vi "Day 2 - Rock Paper Scissors.vi"() -> ()   [LabVIEW 2020, in "AoC 2022.lvlib"]
uses:
  AoC 2022.lvlib
panel:
  out "Puzzle Part-2 Answer":string
  out "Puzzle Answer":string
  in  "Puzzle Input":string
  # "Enter the Puzzle Input and run the VI"
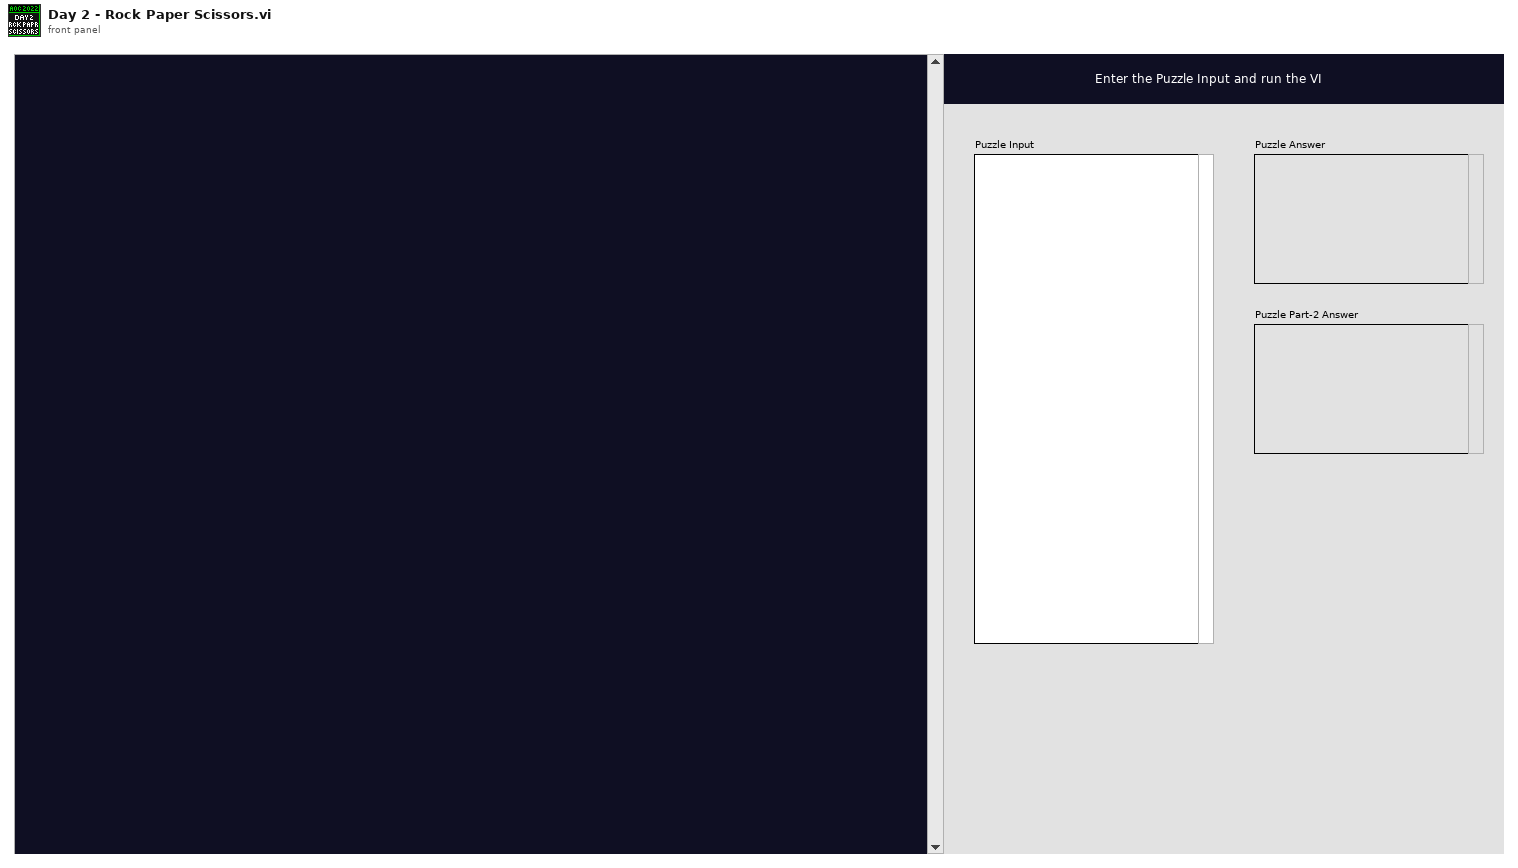
[diagram p1: front panel]
types:
  T1 = typedef "AoC 2022.lvlib/Play Item.ctl" = enum16{"Rock", "Paper", "Scissor"}
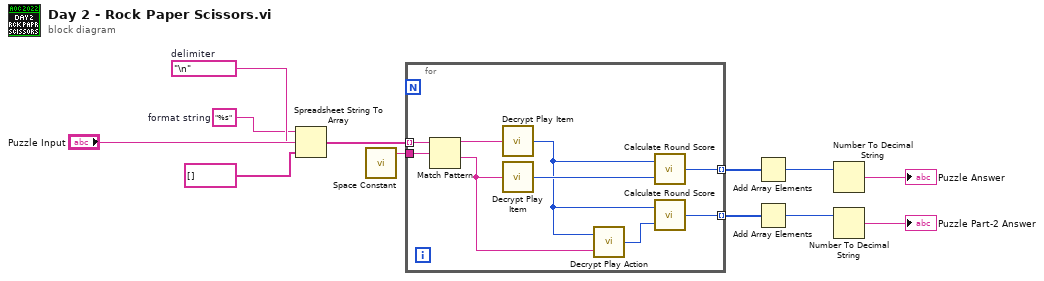
[diagram p0: block diagram]
diagram:
  w10 = "%s"  # format string
  w11 = "\n"  # delimiter
  n1 = Spreadsheet String To Array(delimiter (Tab)=w11, format string=w10, spreadsheet string="Puzzle Input", array type (2D Dbl)=string[] []) -> (array=w8:string[])
  n2 = call <vilib>:"Space Constant.vi"() -> ("String"=w7:string)
  n3 = for {
    tunnel: w8 -> [w21] mode=indexing
    tunnel: w7 -> [w20]
    tunnel: [w17] -> w6 mode=indexing
    tunnel: [w13] -> w2 mode=indexing
    n4 = Match Pattern(string=w21, regular expression=w20) -> (before substring=w19:string, after substring=w16:string)  [unwired: 1 in, 2 out]
    n5 = call "Decrypt Play Item.vi"("Encrypted Play Item"=w19) -> ("Play Item"=w15:T1)  [unwired: 4 in]
    n6 = call "Decrypt Play Item.vi"("Encrypted Play Item"=w16) -> ("Play Item"=w18:T1)  [unwired: 4 in]
    n7 = call "Decrypt Play Action.vi"("Encrypted Play Action"=w16, "Opponent's Move"=w15) -> ("My Move"=w14:T1)
    n8 = call "Calculate Round Score.vi"("My Move"=w18, "Opponent's Move"=w15) -> ("Round Score"=w17:u32)
    n9 = call "Calculate Round Score.vi"("My Move"=w14, "Opponent's Move"=w15) -> ("Round Score"=w13:u32)
  }
  n10 = Add Array Elements(numeric array=w6) -> (sum=w5:u32)
  n11 = Add Array Elements(numeric array=w2) -> (sum=w3:u32)
  n12 = Number To Decimal String(number=w5) -> (decimal integer string=→"Puzzle Answer":string)  [unwired: 1 in]
  n13 = Number To Decimal String(number=w3) -> (decimal integer string=→"Puzzle Part-2 Answer":string)  [unwired: 1 in]
